vi "TT (Main).vi"(7 "Name of Parent Panel":string="Main.vi", 9 "New Center Coords":T1={"Horizontal"=470, "Vertical"=200}, 10 "Config":variant, 11 "Main UI Message Queue":refnum<queue>) -> ()   [LabVIEW 2018, in "TT Module.lvlib"]
doc: "This Continuous Measurement sample project is based on the Queued Message Handler template.\n\nThe Event Handling Loop generates messages based on user interface actions.\n\nThe Message Handling Loop processes messages generated by the Event Handling Loop, or by other messages. There are also Acquisition and Logging message handling loop subVIs, and a chart updating loop."
uses:
  TT Module.lvlib
  support/Message Queue/Message Cluster.ctl
  <vilib>/Utility/miscctls.llb/LVPoint32TypeDef.ctl
  Controls/TT Module Config Cluster.ctl
  Tag VIs/Numeric Alarm Settings Cluster.ctl
  Tag VIs/Tag FGV Operation Enum.ctl
  support/Message Queue/Enqueue Message (Single).vi
  support/User Event - Stop/User Event - Stop.lvlib
  support/Support Library.lvlib
  support/Message Queue/Message Queue.lvlib
  Shared Variables/Dynamic Shared Variables.lvlib
  subVIs/TT Settings Dialog.vi
  support/Command Log VIs/Command Logging.lvlib
  Report Generation/Report Generation.lvlib
panel:
  in  "Settings":bool
  out "Display Cluster":cluster{"Tag Name":string, "Temperature":dbl} {"Temperature" format="%.1f"}
  out "H/W":dbl
  out "Original Height":u32
  out "Original Width":u32
  in  "Start":bool
  in  "Stop":bool
  out "Status":string
  in  "Exit":bool
  out "Input Channel Tag Name":string
  out "Log File path":path
  in  "Force Trigger":bool
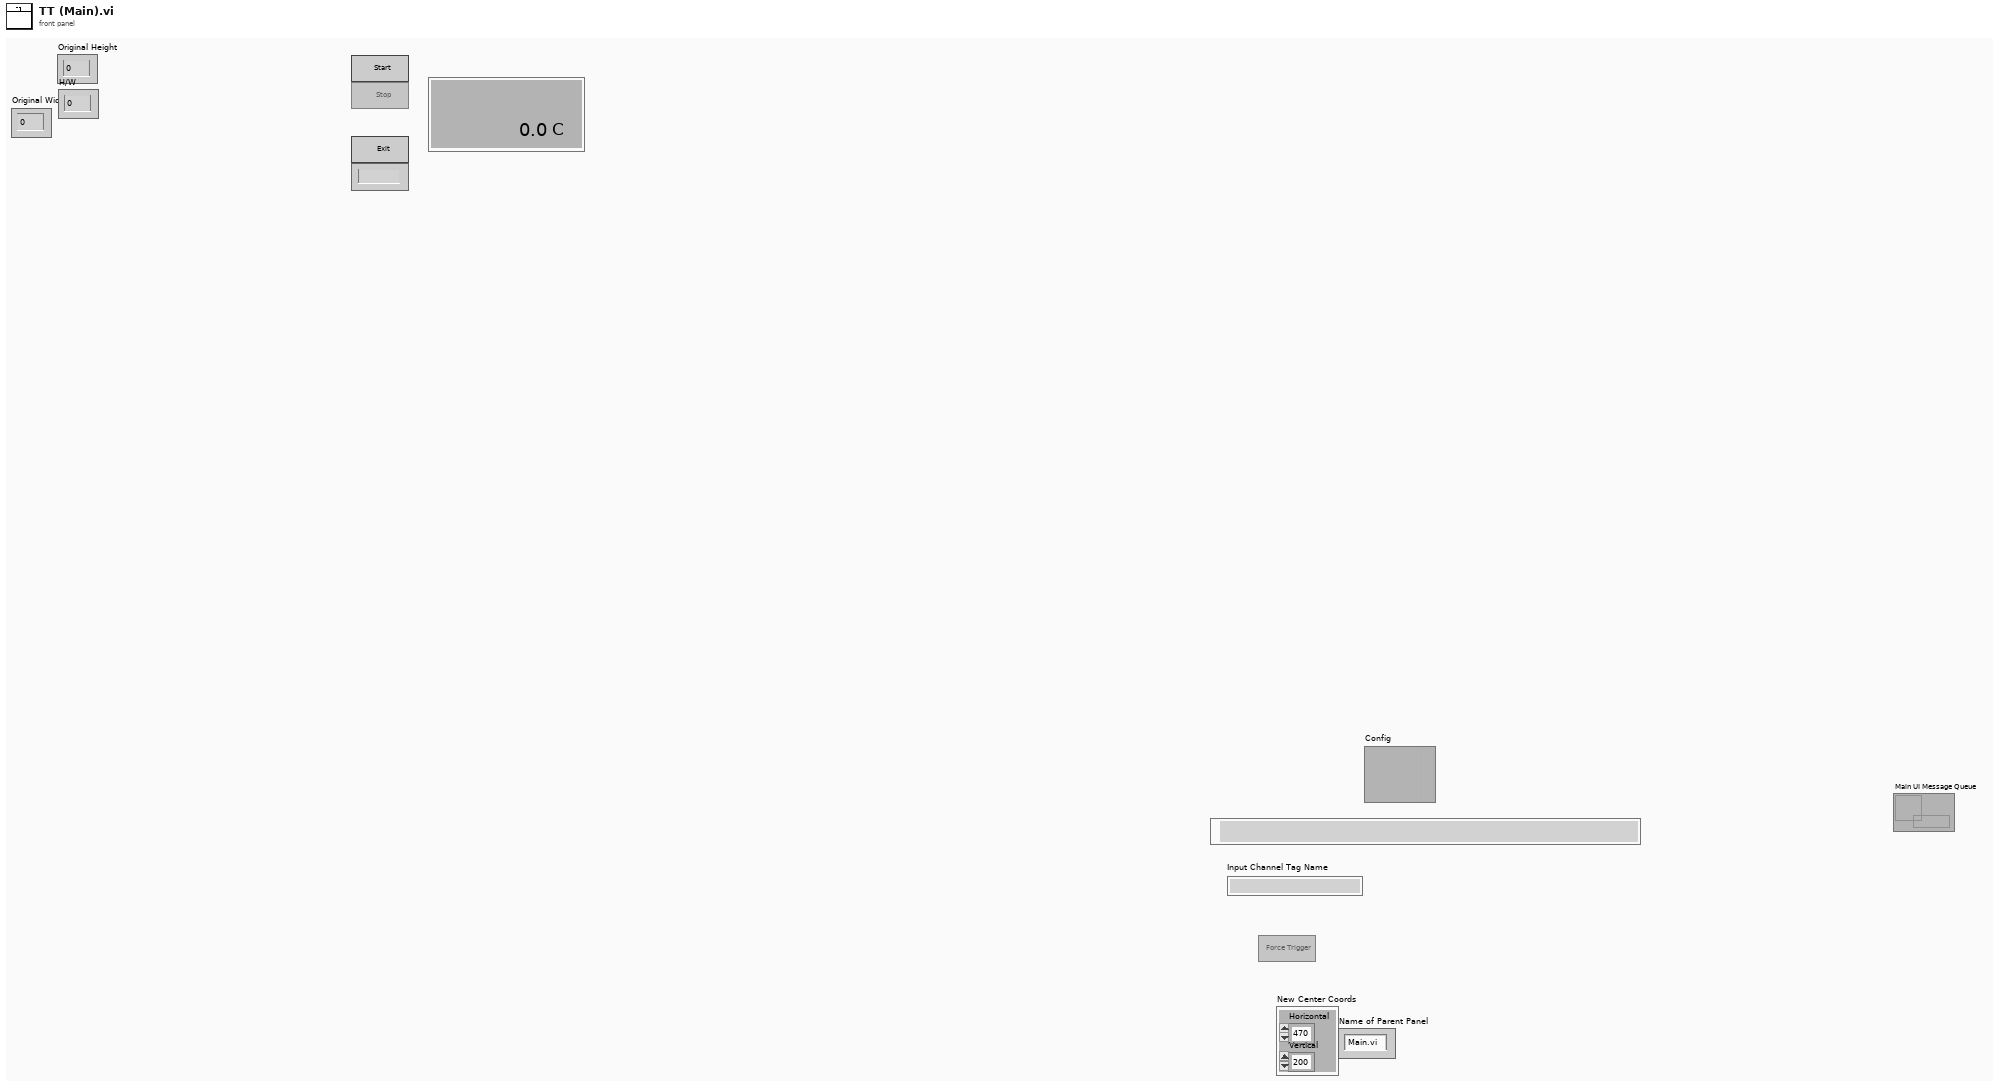
[diagram p1: front panel]
types:
  T1 = typedef "LVPoint32TypeDef.ctl" = cluster{"Horizontal":i32, "Vertical":i32}
  T2 = enum32{"Invalid", "Default", "Floating", "Floating/Auto-Hide", "Modal"}
  T3 = typedef "TT Module.lvlib/TT Module Config Cluster.ctl" = cluster{"GUID":string, "Drop Coords":T1, "Input Channel Tag Name ":string, "Process Name":string, "User name":string, "Queue Name":string, "Input Channel Numeric Alarm Settings":T4[]}
  T4 = typedef "Numeric Alarm Settings Cluster.ctl" = cluster{"enable? (F)":bool, "name":string, "alarm type":enum16{"HI_HI", "HI", "LO", "LO_LO"}, "level/change":dbl, "deadband/time":dbl, "alarm delay":dbl, "priority":u32, "ack type":enum16{"Auto", "User", "None", "Each Occurrence"}, "area":string, "description":string, "log? (T)":bool}
  T5 = typedef "LVPointTypeDef.ctl" = cluster{"Horizontal":i16, "Vertical":i16}
  T6 = typedef "Tag FGV Operation Enum.ctl" = enum16{"Init", "Set Notification Queue", "Create Tag", "Commit", "Write Tag (Numeric)", "Write Tag (Boolean)", "Read All Tags", "Read One Tag", "Delete Tag Category", "Set Alarm Parameters (Numeric)", "Set Alarm Parameters (Boolean)", "Enable All Alarms", "Disable All Alarms", "Delete All Tags", "Read Alarms", "Ack Alarm", "Read Alarm Parameters (Numeric)", "Read Alarm Parameters (Boolean)"}
  T7 = typedef "LVRectTypeDef.ctl" = cluster{"Left":i16, "Top":i16, "Right":i16, "Bottom":i16}
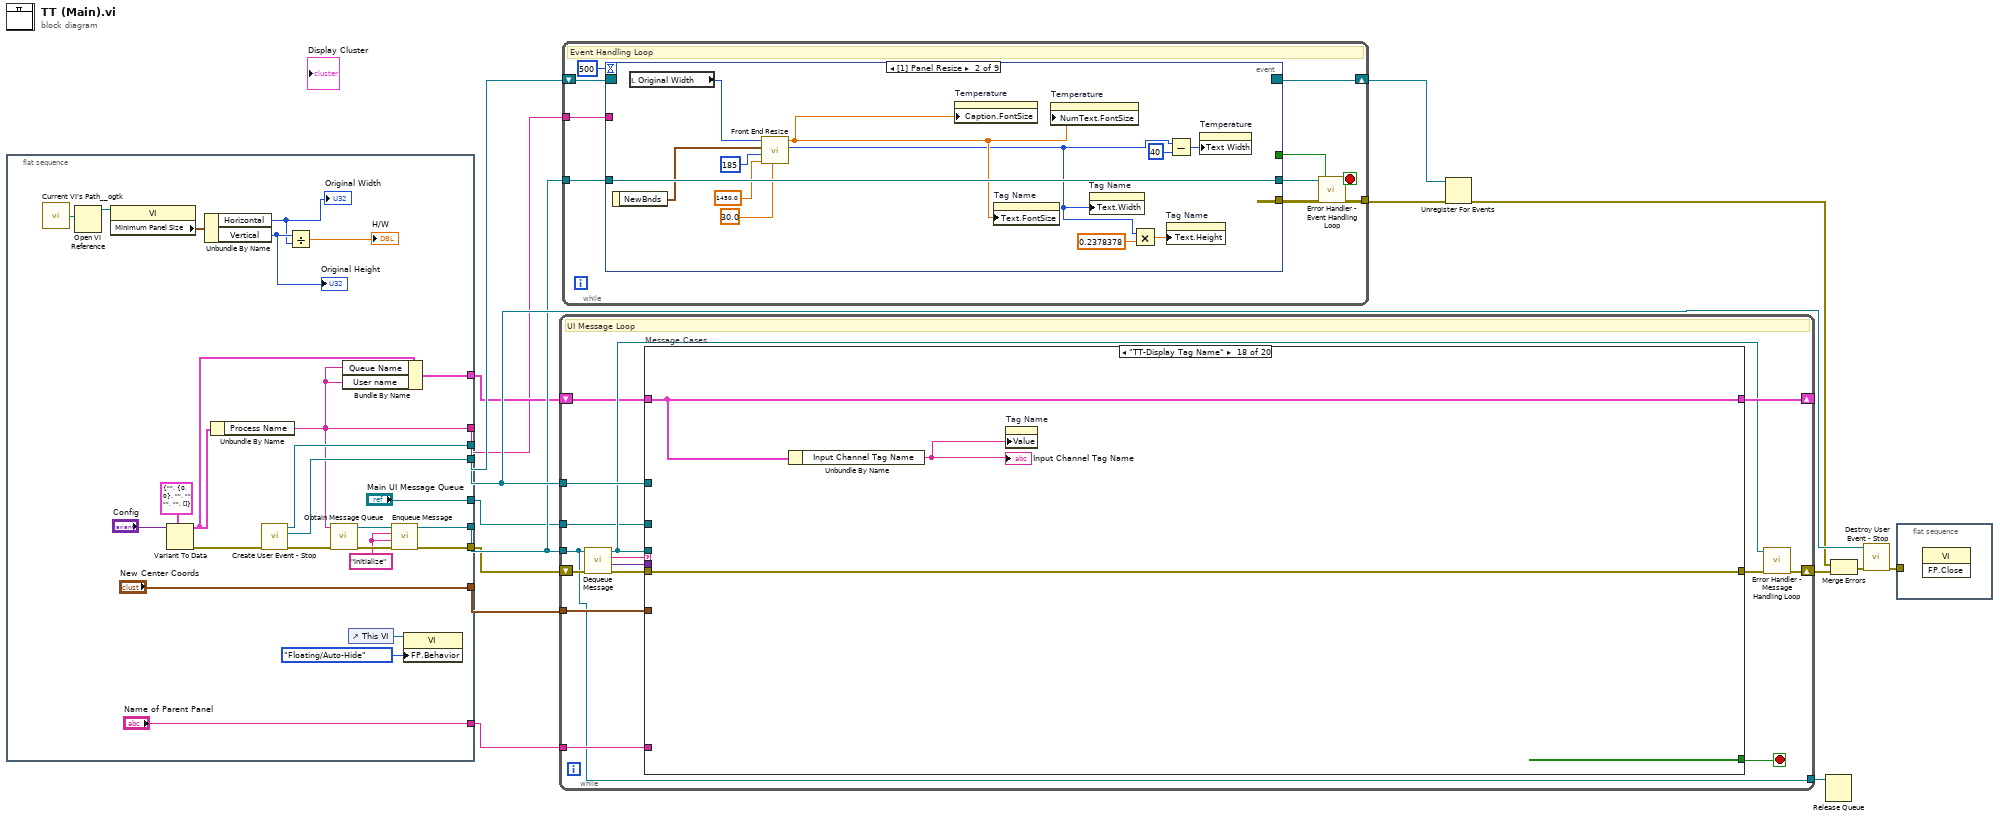
[diagram p0: block diagram]
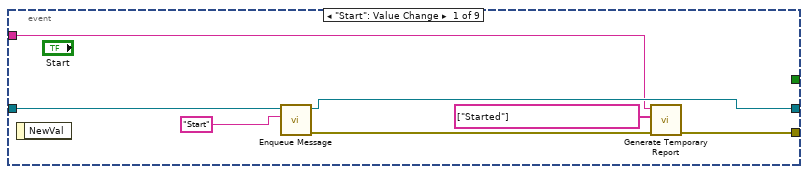
[diagram p2: hidden frame]
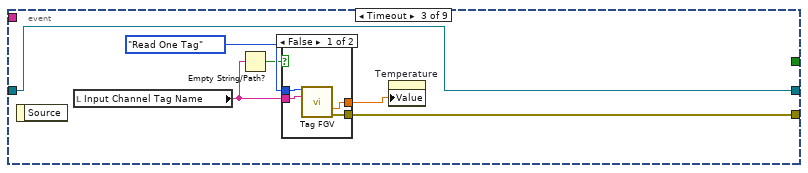
[diagram p3: hidden frame]
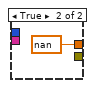
[diagram p4: hidden frame]
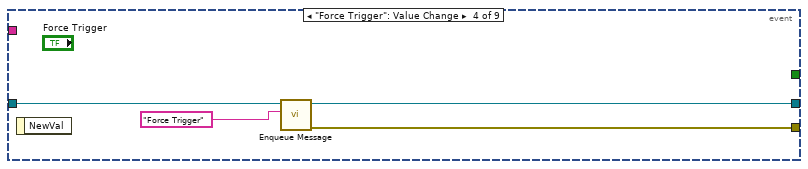
[diagram p5: hidden frame]
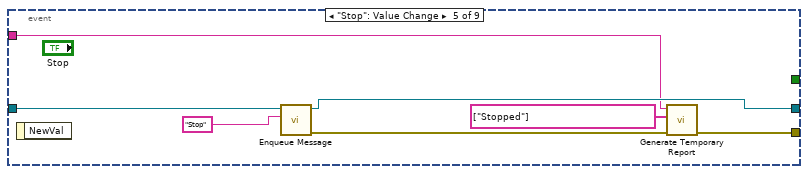
[diagram p6: hidden frame]
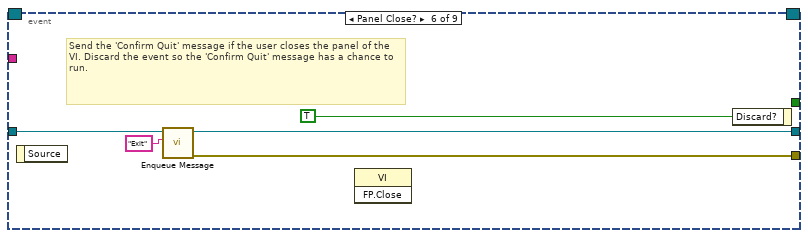
[diagram p7: hidden frame]
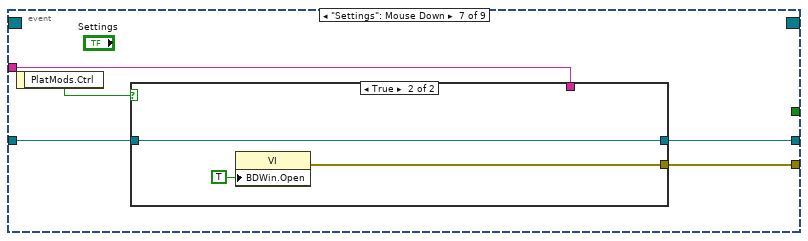
[diagram p8: hidden frame]
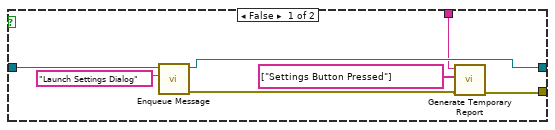
[diagram p9: hidden frame]
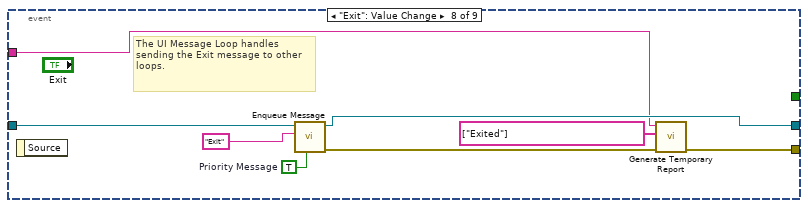
[diagram p10: hidden frame]
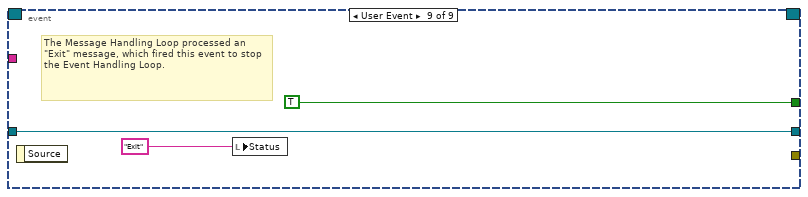
[diagram p11: hidden frame]
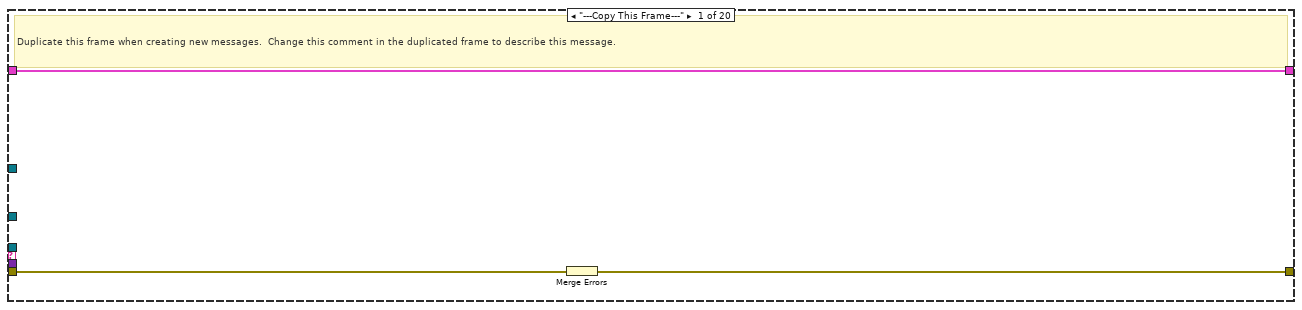
[diagram p12: hidden frame]
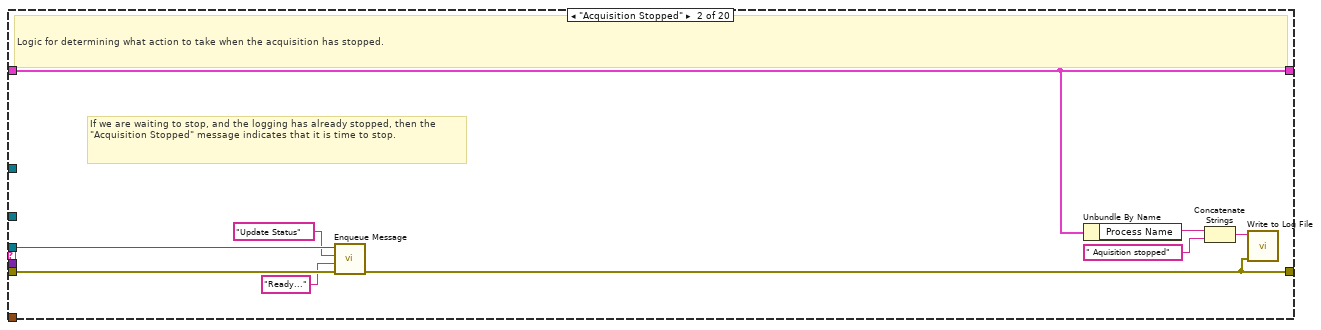
[diagram p13: hidden frame]
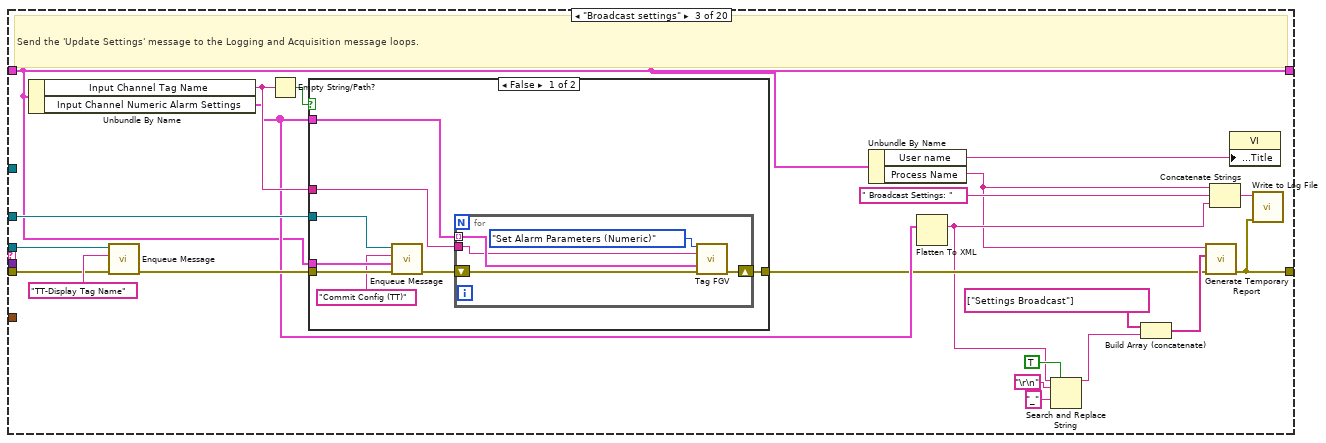
[diagram p14: hidden frame]
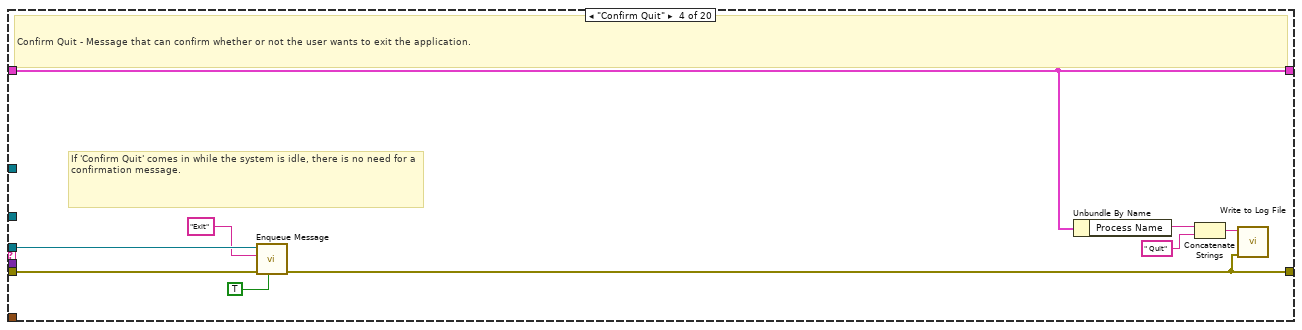
[diagram p16: hidden frame]
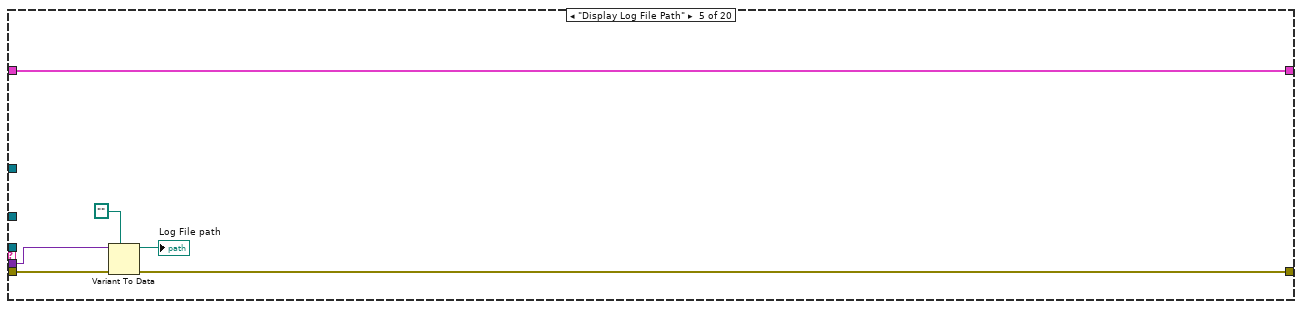
[diagram p17: hidden frame]
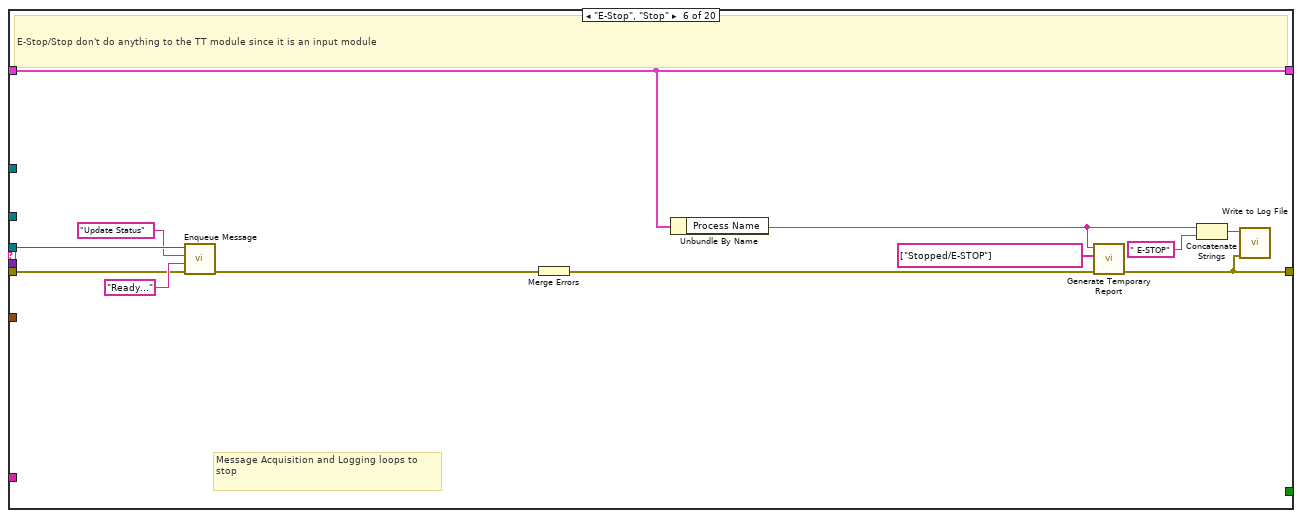
[diagram p18: hidden frame]
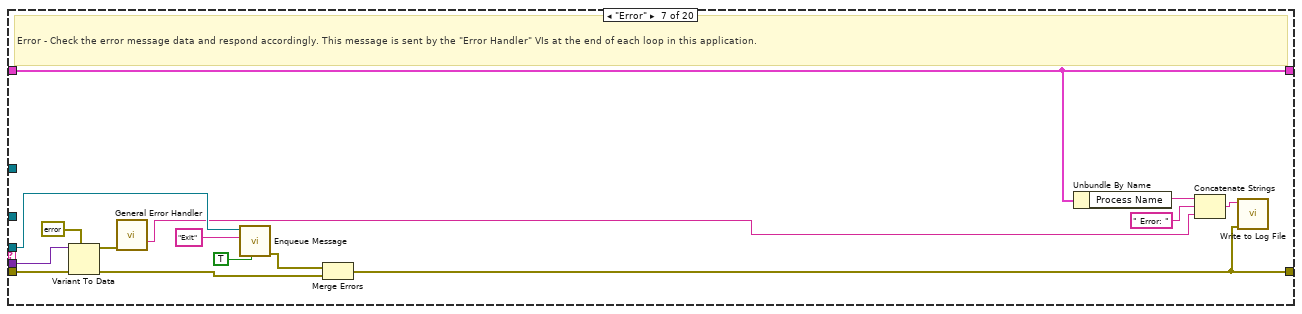
[diagram p19: hidden frame]
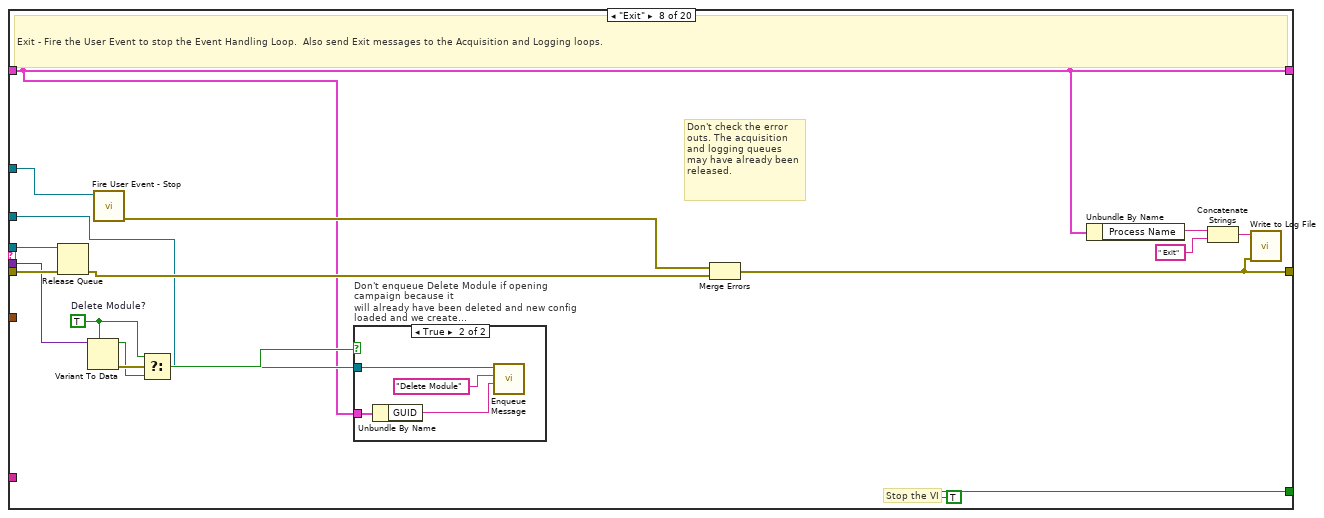
[diagram p20: hidden frame]
diagram:
  n1 = flat-sequence {
    tunnel: [w41] -> w13
    tunnel: [w40] -> w12
    tunnel: [w37] -> w9
    tunnel: [w35] -> w8
    tunnel: ["Main UI Message Queue"] -> w7
    tunnel: ["New Center Coords"] -> w6
    tunnel: ["Name of Parent Panel"] -> w5
    tunnel: [w26] -> w3
    tunnel: [w23] -> w1
    frame #0 {
      w36 = "Initialize" ("Message")
      n2 = call <userlib>:"Current VI's Path__ogtk.vi"() -> ("Current VI's Path (+ Relative)"=w18:path)  [unwired: 1 in]
      n3 = Open VI Reference(vi path=w18) -> (vi reference=w19:refnum<vi>)  [unwired: 5 in, 1 out]
      n4 = property class="VI"(reference=w19) -> ("Minimum Panel Size"=w20:T5)  [unwired: 1 in, 2 out]
      n5 = Variant To Data(type=T3 {"GUID"="", "Drop Coords"={"Horizontal"=0, "Vertical"=0}, "Input Channel Tag Name "="", "Process Name"="", "User name"="", "Queue Name"="", "Input Channel Numeric Alarm Settings"=[]} ("TT Module Config"), Variant="Config") -> (data=w27:T3, error out=w30:errorcluster)  [unwired: 1 in]
      n6 = Unbundle By Name(w20) -> ("Horizontal"=w21:i16, "Vertical"=w22:i16)
      "Original Width" <- w21
      "Original Height" <- w22
      n7 = Unbundle By Name(w27) -> ("Process Name"=w23:string)
      n8 = call "Create User Event - Stop.vi"("error in (no error)"=w30) -> ("error out"=w34:errorcluster, "User Event - Stop"=w40:refnum<user-event>, "Stop Event Registration Refnum"=w41:refnum<event-registration>)  [unwired: 8 in]
      n9 = Divide(x=w22, y=w21) -> (x/y=→"H/W":dbl)
      n10 = call "Obtain Message Queue.vi"("error in (no error)"=w34, "name (unnamed)"=w23) -> ("error out"=w39:errorcluster, "Message Queue"=w38:refnum<queue>)  [unwired: 8 in]
      n11 = Bundle By Name(cluster=w27, "Queue Name"=w23, "User name"=w23) -> (w26:T3)
      n12 = control-ref of="This VI"() -> (w25:refnum<vi>)
      n13 = call-poly "Enqueue Message.vi"("error in (no error)"=w39, "Message Data"=w36, "Message"=w36, "Message Queue"=w38) -> ("error out"=w35:errorcluster, "dup Message Queue"=w37:refnum<queue>)  [unwired: 6 in]
      n14 = property class="VI"(reference=w25, "FP.Behavior"=T2."Floating/Auto-Hide" ("Front Panel Window:Behavior")) -> ()  [unwired: 1 in, 2 out]
    }
  }
  n15 = while {
    tunnel: w9 -> [w42]
    tunnel: w12 -> [w55]
    shift-right: [w48] -> w16
    shift-left: w8 -> [w54]
    shift-right: [w50] -> _
    shift-left: w3 -> [w46]
    tunnel: w7 -> [w45]
    tunnel: w6 -> [w44]
    tunnel: w5 -> [w43]
    tunnel: [w42] -> w2
    stop <- w56 stop-if-true
    # "UI Message Loop"
    n16 = call "Dequeue Message.vi"("error in (no error)"=w54, "Message Queue"=w42) -> ("error out"=w53:errorcluster, "Message Data"=w51:variant, "Message"=w52:string, "dup Message Queue"=w47:refnum<queue>)  [unwired: 6 in]
    n17 = case "Message Cases" shown="\"TT-Display Tag Name\"" w52 {
      selector: w52 -> [_ _ _ _ _ _ _ _ _ _ _ _ _ _ _ _ _ _ _ w266]
      tunnel: w47 -> [_ w67 w90 w113 _ w131 w142 w159 _ _ w197 w209 _ _ w237 _ _ _ _ _]
      tunnel: w53 -> [w59 w68 w88 w112 w114 w128 w146 w162 w168 w181 w194 w211 w218 w224 w235 w243 w253 w256 w263 _]
      tunnel: [w58 w61 w73 w106 w115 w120 w134 w148 w170 w181 w186 w203 w218 w227 w231 w242 w248 w256 w264 w265] -> w49
      tunnel: [_ _ _ _ _ _ _ TRUE _ _ _ _ _ _ _ _ _ _ _ _] -> w56
      tunnel: w51 -> [_ _ _ _ w117 _ w145 w153 _ _ _ _ _ w225 _ _ _ _ w262 _]
      tunnel: w55 -> [_ _ _ _ _ _ _ w161 _ _ _ _ _ _ _ _ _ _ _ _]
      tunnel: [w57 w60 w69 w105 w119 w124 w133 w147 w169 w180 w183 w202 w219 w229 w230 w245 w247 w257 w259 w271] -> w50
      tunnel: w46 -> [w57 w60 w69 w105 w119 w124 w133 w147 w169 w180 w183 w207 w219 w229 w230 w245 w247 w257 w259 w271]
      tunnel: w45 -> [_ _ w85 _ _ _ _ w152 _ _ _ _ _ _ _ _ w252 _ _ _]
      tunnel: w44 -> [_ _ _ _ _ _ _ _ _ _ w191 _ _ _ _ _ _ _ _ _]
      tunnel: w43 -> [_ _ _ _ _ _ _ _ _ _ w189 _ _ _ _ _ _ _ _ _]
      frame "---Copy This Frame---" {
        # "Duplicate this frame when creating new messages.  Change this comment in the duplicated frame to describe this message."
        n18 = Merge Errors(w59) -> (w58:errorcluster)
      }
      frame "Acquisition Stopped" {
        # "If we are waiting to stop, and the logging has already stopped, then the \"Acquisition Stopped\" message indicates that it is time to stop."
        # "Logic for determining what action to take when the acquisition has stopped."
        n19 = call-poly "Enqueue Message.vi"("error in (no error)"=w68, "Message Data"="Ready..." ("Message"), "Message"="Update Status", "Message Queue"=w67) -> ("error out"=w61:errorcluster)  [unwired: 6 in, 1 out]
        n20 = Unbundle By Name(w60) -> ("Process Name"=w64:string)
        n21 = Concatenate Strings(w64, " Aquisition stopped" ("text")) -> (w63:string)
        n22 = call "Write to Log File.vi"("error in"=w61, "text"=w63) -> ()  [unwired: 9 in, 1 out]
      }
      frame "Broadcast settings" {
        # "Send the 'Update Settings' message to the Logging and Acquisition message loops."
        n23 = Unbundle By Name(w69) -> ("Input Channel Tag Name"=w84:string, "Input Channel Numeric Alarm Settings"=w81:T4[])
        n24 = call-poly "Enqueue Message.vi"("error in (no error)"=w88, "Message"="TT-Display Tag Name", "Message Queue"=w90) -> ("error out"=w86:errorcluster)  [unwired: 7 in, 1 out]
        n25 = Empty String/Path?(string/path=w84) -> (empty?=w87:bool)
        n26 = case shown="False" w87 {
          tunnel: w81 -> [w98 _]
          tunnel: [w97 w104] -> w74
          tunnel: w86 -> [w96 w104]
          tunnel: w69 -> [w95 _]
          tunnel: w85 -> [w94 _]
          tunnel: w84 -> [w92 _]
          frame False {
            n27 = call-poly "Enqueue Message.vi"("error in (no error)"=w96, "Message Data"=w95, "Message"="Commit Config (TT)", "Message Queue"=w94) -> ("error out"=w93:errorcluster)  [unwired: 6 in, 1 out]
            n28 = for {
              tunnel: w98 -> [w102] mode=indexing
              tunnel: w92 -> [w101]
              shift-right: [w99] -> w97
              shift-left: w93 -> [w100]
              n29 = call "Tag FGV.vi"("Operation"=Tag_FGV_Operation_Enum."Set Alarm Parameters (Numeric)", "Tag Name"=w101, "Data"=w102, "error in (no error)"=w100) -> ("error out"=w99:errorcluster)  [unwired: 4 in, 7 out]
            }
          }
          frame True {
          }
        }
        n30 = Unbundle By Name(w69) -> ("User name"=w80:string, "Process Name"=w70:string)
        n31 = Flatten To XML(anything=w81) -> (xml string=w72:string)
        n32 = Search and Replace String(replace all?=TRUE ("replace all? (F)"), input string=w72, search string="\r\n", replace string="_" ("replace string (\"\")")) -> (result string=w71:string)  [unwired: 4 in, 3 out]
        n33 = Build Array (concatenate)(string[] ["Settings Broadcast"] ("Line of Events"), w71) -> (w75:string[])
        n34 = call "Generate Temporary Report.vi"("error in (no error)"=w74, "Line of Events"=w75, "Module Name"=w70) -> ("error out"=w73:errorcluster)  [unwired: 8 in]
        n35 = Concatenate Strings(w70, " Broadcast Settings: " ("text"), w72) -> (w83:string)
        n36 = property class="VI"("Front Panel.Title"=w80) -> ()  [unwired: 2 in, 2 out]
        n37 = call "Write to Log File.vi"("error in"=w73, "text"=w83) -> ()  [unwired: 9 in, 1 out]
      }
      frame "Confirm Quit" {
        # "If 'Confirm Quit' comes in while the system is idle, there is no need for a confirmation message."
        # "Confirm Quit - Message that can confirm whether or not the user wants to exit the application."
        n38 = call-poly "Enqueue Message.vi"("Priority Message? (F)"=TRUE, "error in (no error)"=w112, "Message"="Exit", "Message Queue"=w113) -> ("error out"=w106:errorcluster)  [unwired: 6 in, 1 out]
        n39 = Unbundle By Name(w105) -> ("Process Name"=w109:string)
        n40 = Concatenate Strings(w109, " Quit" ("text")) -> (w108:string)
        n41 = call "Write to Log File.vi"("error in"=w106, "text"=w108) -> ()  [unwired: 9 in, 1 out]
      }
      frame "Display Log File Path" {
        n42 = Variant To Data(error in=w114, type=path "", Variant=w117) -> (data=→"Log File path":path, error out=w115:errorcluster)
      }
      frame "E-Stop", "Stop" {
        # "Message Acquisition and Logging loops to stop"
        # "E-Stop/Stop don't do anything to the TT module since it is an input module"
        n43 = call-poly "Enqueue Message.vi"("error in (no error)"=w128, "Message Data"="Ready..." ("Ready..."), "Message"="Update Status", "Message Queue"=w131) -> ("error out"=w127:errorcluster)  [unwired: 6 in, 1 out]
        n44 = Merge Errors(w127) -> (w121:errorcluster)
        n45 = Unbundle By Name(w124) -> ("Process Name"=w122:string)
        n46 = call "Generate Temporary Report.vi"("error in (no error)"=w121, "Line of Events"=string[] ["Stopped/E-STOP"], "Module Name"=w122) -> ("error out"=w120:errorcluster)  [unwired: 8 in]
        n47 = Concatenate Strings(w122, " E-STOP" ("text")) -> (w126:string)
        n48 = call "Write to Log File.vi"("error in"=w120, "text"=w126) -> ()  [unwired: 9 in, 1 out]
      }
      frame "Error" {
        # "Error - Check the error message data and respond accordingly. This message is sent by the \"Error Handler\" VIs at the end of each loop in this application."
        n49 = Variant To Data(error in=w146, type=errorcluster {"status"=FALSE, "code"=0, "source"=""} ("error out"), Variant=w145) -> (data=w143:errorcluster, error out=w139:errorcluster)
        n50 = call <vilib>:"General Error Handler.vi"("error in (no error)"=w143) -> ("message"=w132:string)  [unwired: 10 in, 4 out]
        n51 = call-poly "Enqueue Message.vi"("Priority Message? (F)"=TRUE, "Message"="Exit", "Message Queue"=w142) -> ("error out"=w138:errorcluster)  [unwired: 7 in, 1 out]
        n52 = Merge Errors(w138, w139) -> (w134:errorcluster)
        n53 = Unbundle By Name(w133) -> ("Process Name"=w137:string)
        n54 = Concatenate Strings(w137, " Error: " ("text"), w132) -> (w136:string)
        n55 = call "Write to Log File.vi"("error in"=w134, "text"=w136) -> ()  [unwired: 9 in, 1 out]
      }
      frame "Exit" {
        w156 = TRUE  # Delete Module?
        # "Don't check the error outs. The acquisition and logging queues may have already been released."
        # "Stop the VI"
        # "Exit - Fire the User Event to stop the Event Handling Loop.  Also send Exit messages to the Acquisition and Logging loops."
        n56 = Release Queue(queue=w159, error in (no error)=w162) -> (error out=w158:errorcluster)  [unwired: 1 in, 2 out]
        n57 = Variant To Data(type=w156, Variant=w153) -> (data=w155:bool, error out=w157:errorcluster)  [unwired: 1 in]
        n58 = call "Fire User Event - Stop.vi"("User Event - Stop"=w161) -> ("error out"=w160:errorcluster)  [unwired: 10 in]
        n59 = Select(t=w156, s=w157, f=w155) -> (s? t:f=w154:bool)
        n60 = case "Don't enqueue Delete Module if opening campaign because it\nwill already have been deleted and new config loaded and we create\na race condition." shown="True" w154 {
          tunnel: w152 -> [_ w166]
          tunnel: w147 -> [_ w165]
          frame False {
          }
          frame True {
            n61 = Unbundle By Name(w165) -> ("GUID"=w164:string)
            n62 = call-poly "Enqueue Message.vi"("Message Data"=w164, "Message"="Delete Module", "Message Queue"=w166) -> ()  [unwired: 7 in, 2 out]
          }
        }
        n63 = Merge Errors(w160, w158) -> (w148:errorcluster)
        n64 = Unbundle By Name(w147) -> ("Process Name"=w151:string)
        n65 = Concatenate Strings(w151, " Exit" ("text")) -> (w150:string)
        n66 = call "Write to Log File.vi"("error in"=w148, "text"=w150) -> ()  [unwired: 9 in, 1 out]
      }
      frame "Force Trigger" {
        # "Force Trigger - send a message to the Logging message loop to start logging."
        n67 = Merge Errors(w168) -> (w170:errorcluster)
      }
      frame "Init UI Refs" {
        # "Init UI Refs - Store control references for UI controls.  Also enable/disable controls appropriately."
        n68 = control-ref of="Exit"() -> (w174:refnum<vi>)
        n69 = control-ref of="Start"() -> (w177:refnum<vi>)
        n70 = property class="VI"("Front Panel.Closeable"=TRUE ("Front Panel Window:Closeable")) -> ()  [unwired: 2 in, 2 out]
        n71 = Build Array(w174, w177) -> (w176:refnum<vi>[])
        n72 = call "Set Enable State on Multiple Controls.vi"("Enable?"=TRUE, "Controls"=w176) -> ()  [unwired: 10 in]
        n73 = control-ref of="Force Trigger"() -> (w173:refnum<vi>)
        n74 = control-ref of="Stop"() -> (w172:refnum<vi>)
        n75 = Build Array(w172, w173) -> (w171:refnum<vi>[])
        n76 = control-ref of="Status"() -> ()  [unwired: 1 out]
        n77 = call "Set Enable State on Multiple Controls.vi"("Enable?"=FALSE, "Controls"=w171) -> ()  [unwired: 10 in]
      }
      frame "Initialize" {
        # "Initialize - Get configuration settings, then message the UI to initialize, and broadcast the settings to the other message loops."
        n78 = Unbundle By Name(w183) -> ("Process Name"=w182:string)
        n79 = property class="VI" props=["FP.State"]() -> (reference out=w190:refnum<vi>)  [unwired: 2 in, 2 out]
        n80 = call-poly "Enqueue Message.vi"("error in (no error)"=w194, "Message"="Init UI Refs", "Message Queue"=w197) -> ("error out"=w195:errorcluster, "dup Message Queue"=w196:refnum<queue>)  [unwired: 7 in]
        n81 = call "Make Child and Move.vi"("Process Name"=w182, "Name of Parent Panel"=w189, "New Center Coords"=w191, "VI in"=w190) -> ()  [unwired: 8 in]
        n82 = call-poly "Enqueue Message.vi"("error in (no error)"=w195, "Message"="Broadcast Settings", "Message Queue"=w196) -> ("error out"=w192:errorcluster, "dup Message Queue"=w193:refnum<queue>)  [unwired: 7 in]
        n83 = call-poly "Enqueue Message.vi"("error in (no error)"=w192, "Message Data"="Ready..." ("Ready..."), "Message"="Update Status", "Message Queue"=w193) -> ("error out"=w186:errorcluster)  [unwired: 6 in, 1 out]
        n84 = Unbundle By Name(w183) -> ("Process Name"=w184:string)
        n85 = call "Generate Temporary Report.vi"("Line of Events"=string[] ["Initialized"], "Module Name"=w184) -> ()  [unwired: 9 in, 1 out]
        n86 = Concatenate Strings(w184, " Initialize" ("text")) -> (w188:string)
        n87 = call "Write to Log File.vi"("error in"=w186, "text"=w188) -> ()  [unwired: 9 in, 1 out]
      }
      frame "Launch Settings Dialog" {
        # "Launch the Settings Dialog when the user clicks the 'Settings' button."
        n88 = call-by-ref "?"("error in (no error)"=w211, "TT Module Config in"=w207) -> ("error out"=w208:errorcluster, "Cancelled?"=w210:bool, "TT Module Config out"=w202:T3)  [unwired: 8 in, 3 out]
        n89 = case shown="False" w210 {
          tunnel: w209 -> [w212 _]
          tunnel: w208 -> [w213 w217]
          tunnel: [w216 w217] -> w203
          tunnel: w202 -> [w214 _]
          frame False {
            n90 = call-poly "Enqueue Message.vi"("error in (no error)"=w213, "Message Data"=w214, "Message"="Broadcast Settings", "Message Queue"=w212) -> ("error out"=w216:errorcluster)  [unwired: 6 in, 1 out]
          }
          frame True {
          }
        }
        n91 = Unbundle By Name(w202) -> ("Process Name"=w206:string)
        n92 = Concatenate Strings(w206, " Settings Dialog Launched" ("text")) -> (w205:string)
        n93 = call "Write to Log File.vi"("error in"=w203, "text"=w205) -> ()  [unwired: 9 in, 1 out]
      }
      frame "Logging Stopped" {
        # "Logic for determining what action to take when the logging has stopped."
      }
      frame "Send to Sequence" {
        n94 = Variant To Data(error in=w224, type=refnum<queue> refnum ("Message Queue"), Variant=w225) -> (data=w223:refnum<queue>, error out=w222:errorcluster)
        n95 = local read "Display Cluster"() -> (w221:cluster{"Tag Name":string, "Temperature":dbl})
        n96 = Unbundle By Name(w221) -> ("Temperature"=w220:dbl)
        n97 = call-poly "Enqueue Message.vi"("error in (no error)"=w222, "Message Data"=w220, "Message"="Sent to Sequence", "Message Queue"=w223) -> ("error out"=w227:errorcluster)  [unwired: 6 in, 1 out]
      }
      frame "Start" {
        # "Message Acquisition and Logging loops to start"
        # "Start - The action starts from the DAQ VI not the TT module"
        n98 = call-poly "Enqueue Message.vi"("error in (no error)"=w235, "Message"="Broadcast settings", "Message Queue"=w237) -> ("error out"=w238:errorcluster, "dup Message Queue"=w236:refnum<queue>)  [unwired: 7 in]
        n99 = call-poly "Enqueue Message.vi"("error in (no error)"=w238, "Message"="Start Loops", "Message Queue"=w236) -> ("error out"=w239:errorcluster)  [unwired: 7 in, 1 out]
        n100 = Merge Errors(w239) -> (w231:errorcluster)
        n101 = Unbundle By Name(w230) -> ("Process Name"=w234:string)
        n102 = Concatenate Strings(w234, " Start" ("text")) -> (w233:string)
        n103 = call "Write to Log File.vi"("error in"=w231, "text"=w233) -> ()  [unwired: 9 in, 1 out]
      }
      frame "Start Loops" {
        # "Message Acquisition and Logging loops to start"
        # "Start - DAQ VI Handles this"
        n104 = Unbundle By Name(w245) -> ("Process Name"=w244:string)
        n105 = call "Generate Temporary Report.vi"("error in (no error)"=w243, "Line of Events"=string[] ["Started"], "Module Name"=w244) -> ("error out"=w242:errorcluster)  [unwired: 8 in]
      }
      frame "Start Log" {
        # "Message Acquisition and Logging loops to start"
        # "Start Log: The Tags are created in the DAQ vi, but the # of Tags Created messages needs to match the number of modules dropped"
        n106 = call-poly "Enqueue Message.vi"("error in (no error)"=w253, "Message"="Tags Created", "Message Queue"=w252) -> ("error out"=w248:errorcluster)  [unwired: 7 in, 1 out]
        n107 = Unbundle By Name(w247) -> ("Process Name"=w251:string)
        n108 = Concatenate Strings(w251, " Tags Made" ("text")) -> (w250:string)
        n109 = call "Write to Log File.vi"("error in"=w248, "text"=w250) -> ()  [unwired: 9 in, 1 out]
      }
      frame "TT-Display Tag Name" {
        n110 = Unbundle By Name(w257) -> ("Input Channel Tag Name"=w255:string)
        "Input Channel Tag Name" <- w255
        n111 = property on="Tag Name" class="Str"("Value"=w255) -> ()  [unwired: 2 in, 2 out]
      }
      frame "Update Status" {
        # "Update Display - Convert the message data to a string to display in the Status indicator."
        n112 = Variant To Data(error in=w263, type="", Variant=w262) -> (data=→"Status":string, error out=w260:errorcluster)
        n113 = Merge Errors(w260) -> (w264:errorcluster)
      }
      frame Default {
        # "'Default' case only runs if there is a message that isn't defined in any of the other cases.  Output a programming error."
        n114 = Concatenate Strings("The invalid message string " ("string"), w266, " was received in TT Main." ("string")) -> (w267:string)
        n115 = Bundle By Name(cluster=errorcluster {"status"=TRUE, "code"=1, "source"=""} ("error constant"), "source"=w267) -> (w265:errorcluster)
        n116 = Unbundle By Name(w271) -> ("Process Name"=w274:string)
        n117 = Concatenate Strings(w274, " Incorrect Message Received: " ("text"), w266) -> (w273:string)
        n118 = call "Write to Log File.vi"("error in"=w265, "text"=w273) -> ()  [unwired: 9 in, 1 out]
      }
    }
    n119 = call "Error Handler - Message Handling Loop.vi"("error in (no error)"=w49, "Message Queue"=w47) -> ("dup error in"=w48:errorcluster)  [unwired: 8 in, 1 out]
  }
  n120 = while {
    tunnel: w9 -> [w282]
    tunnel: [w277] -> w15
    shift-right: [w281] -> w10
    shift-left: w13 -> [w283]
    tunnel: w1 -> [w275]
    stop <- w280 stop-if-true
    # "Event Handling Loop"
    n121 = event shown="[1] Panel Resize" {
      selector: w283 -> [_ _ _ _ _ _ _ _ _]
      dyn-events: [_ _ _ _ _ _ _ _ _] -> w281
      timeout: 500 -> [_ _ _ _ _ _ _ _ _]
      tunnel: [_ _ _ _ _ _ _ _ TRUE ("Discard?")] -> w280
      tunnel: w282 -> [w289 w302 w304 w316 w323 w327 w333 w350 w353]
      tunnel: [w284 _ w307 w315 w318 w325 w334 w345 _] -> w278
      tunnel: [w288 w302 w304 w314 w322 w326 w332 w349 w353] -> w279
      tunnel: w275 -> [w285 _ _ _ w319 _ w330 w347 _]
      event "Start": Value Change {
        n122 = event-data() -> ()  [unwired: 1 in, 1 out]
        n123 = call-poly "Enqueue Message.vi"("Message"="Start", "Message Queue"=w289) -> ("error out"=w286:errorcluster, "dup Message Queue"=w288:refnum<queue>)  [unwired: 8 in]
        n124 = call "Generate Temporary Report.vi"("error in (no error)"=w286, "Line of Events"=string[] ["Started"], "Module Name"=w285) -> ("error out"=w284:errorcluster)  [unwired: 8 in]
      }
      event Panel Resize {
        n125 = event-data() -> ("NewBnds"=w298:T7)  [unwired: 1 in]
        n126 = local read "Original Width"() -> (w297:u32)
        n127 = call "Front End Resize.vi"("Starting Font"=30.0, "Area to Font Division"=1450.0, "Original Text Box Width"=185, "NewBnds"=w298, "Original Panel Width"=w297) -> ("New Text Box Width"=w293:u64, "New Font Size"=w296:dbl)  [unwired: 5 in]
        n128 = property on="Temperature" class="DigNum (strict)"("Caption.FontSize"=w296) -> ()  [unwired: 2 in, 2 out]
        n129 = property on="Tag Name" class="Str"("Text.FontSize"=w296) -> ()  [unwired: 2 in, 2 out]
        n130 = property on="Temperature" class="DigNum (strict)"("NumText.FontSize"=w296) -> ()  [unwired: 2 in, 2 out]
        n131 = property on="Tag Name" class="Str"("Text.Width"=w293) -> ()  [unwired: 2 in, 2 out]
        n132 = Multiply(x=w293, y=0.2378378 ("Starting Font")) -> (x*y=w292:dbl)
        n133 = property on="Tag Name" class="Str"("Text.Height"=w292) -> ()  [unwired: 2 in, 2 out]
        n134 = Subtract(x=w293, y=u64 40) -> (x-y=w295:u64)
        n135 = property on="Temperature" class="DigNum (strict)"("Text Width"=w295) -> ()  [unwired: 2 in, 2 out]
      }
      event Timeout {
        n136 = event-data() -> ()  [unwired: 1 in, 1 out]
        n137 = local read "Input Channel Tag Name"() -> (w306:string)
        n138 = Empty String/Path?(string/path=w306) -> (empty?=w305:bool)
        n139 = case shown="False" w305 {
          tunnel: Tag_FGV_Operation_Enum."Read One Tag" ("Operation") -> [w312 _]
          tunnel: [w311 nan ("Tag Value")] -> w303
          tunnel: [w310 _] -> w307
          tunnel: w306 -> [w309 _]
          frame False {
            n140 = call "Tag FGV.vi"("Operation"=w312, "Tag Name"=w309) -> ("Tag Value"=w311:dbl, "error out"=w310:errorcluster)  [unwired: 6 in, 6 out]
          }
          frame True {
          }
        }
        n141 = property on="Temperature" class="DigNum (strict)"("Value"=w303) -> ()  [unwired: 2 in, 2 out]
      }
      event "Force Trigger": Value Change {
        n142 = event-data() -> ()  [unwired: 1 in, 1 out]
        n143 = call-poly "Enqueue Message.vi"("Message"="Force Trigger", "Message Queue"=w316) -> ("error out"=w315:errorcluster, "dup Message Queue"=w314:refnum<queue>)  [unwired: 8 in]
      }
      event "Stop": Value Change {
        n144 = event-data() -> ()  [unwired: 1 in, 1 out]
        n145 = call-poly "Enqueue Message.vi"("Message"="Stop", "Message Queue"=w323) -> ("error out"=w320:errorcluster, "dup Message Queue"=w322:refnum<queue>)  [unwired: 8 in]
        n146 = call "Generate Temporary Report.vi"("error in (no error)"=w320, "Line of Events"=string[] ["Stopped"], "Module Name"=w319) -> ("error out"=w318:errorcluster)  [unwired: 8 in]
      }
      event Panel Close? {
        # "Send the 'Confirm Quit' message if the user closes the panel of the VI. Discard the event so the 'Confirm Quit' message has a chance to run."
        n147 = event-data() -> ()  [unwired: 1 in, 1 out]
        n148 = call-poly "Enqueue Message.vi"("Message"="Exit", "Message Queue"=w327) -> ("error out"=w325:errorcluster, "dup Message Queue"=w326:refnum<queue>)  [unwired: 8 in]
        n149 = invoke class="VI" method="FP.Close"() -> ()  [unwired: 3 in, 3 out]
        n150 = event-data("Discard?"=TRUE) -> ()  [unwired: 1 in, 1 out]
      }
      event "Settings": Mouse Down {
        n151 = event-data() -> ("PlatMods.Ctrl"=w331:bool)  [unwired: 1 in]
        n152 = case shown="True" w331 {
          tunnel: [w336 w343] -> w334
          tunnel: w333 -> [w340 w342]
          tunnel: [w339 w342] -> w332
          tunnel: w330 -> [w335 _]
          frame False {
            n153 = call-poly "Enqueue Message.vi"("Message"="Launch Settings Dialog", "Message Queue"=w340) -> ("error out"=w337:errorcluster, "dup Message Queue"=w339:refnum<queue>)  [unwired: 8 in]
            n154 = call "Generate Temporary Report.vi"("error in (no error)"=w337, "Line of Events"=string[] ["Settings Button Pressed"], "Module Name"=w335) -> ("error out"=w336:errorcluster)  [unwired: 8 in]
          }
          frame True {
            n155 = property class="VI"("BDWin.Open"=TRUE ("Block Diagram Window:Open")) -> (error out=w343:errorcluster)  [unwired: 2 in, 1 out]
          }
        }
      }
      event "Exit": Value Change {
        w351 = TRUE  # Priority Message
        # "The UI Message Loop handles sending the Exit message to other loops."
        n156 = event-data() -> ()  [unwired: 1 in, 1 out]
        n157 = call-poly "Enqueue Message.vi"("Priority Message? (F)"=w351, "Message"="Exit", "Message Queue"=w350) -> ("error out"=w346:errorcluster, "dup Message Queue"=w349:refnum<queue>)  [unwired: 7 in]
        n158 = call "Generate Temporary Report.vi"("error in (no error)"=w346, "Line of Events"=string[] ["Exited"], "Module Name"=w347) -> ("error out"=w345:errorcluster)  [unwired: 8 in]
      }
      event User Event {
        # "The Message Handling Loop processed an \"Exit\" message, which fired this event to stop the Event Handling Loop."
        n159 = event-data() -> ()  [unwired: 1 in, 1 out]
        n160 = local write "Status"("Exit" ("Exit String")) -> ()
      }
    }
    n161 = call "Error Handler - Event Handling Loop.vi"("error in (no error)"=w278, "Message Queue"=w279) -> ("dup error in"=w277:errorcluster)  [unwired: 8 in, 1 out]
  }
  n162 = Unregister For Events(event registration refnum=w10, error in=w15) -> (error out=w11:errorcluster)
  n163 = Release Queue(queue=w2) -> ()  [unwired: 2 in, 3 out]
  n164 = Merge Errors(w11, w16) -> (w14:errorcluster)
  n165 = call "Destroy User Event - Stop.vi"("error in (no error)"=w14, "User Event - Stop"=w12) -> ("error out"=w4:errorcluster)  [unwired: 9 in]
  n166 = flat-sequence {
    tunnel: w4 -> [_]
    frame #0 {
      n167 = invoke class="VI" method="FP.Close"() -> ()  [unwired: 3 in, 3 out]
    }
  }
